vi "Supervisor MATLAB Write Client.vi"() -> ()   [LabVIEW 2017]
uses:
  <vilib>/OPCUA/controls/Write Status.ctl
  <vilib>/OPCUA/controls/NodeId.ctl
  <vilib>/OPCUA/client/Multiple Write Bool Array.vi
  <vilib>/OPCUA/NI OPC UA Client.lvlib
panel:
  in  "error in (no error)":errorcluster
  in  "Stop MATLAB Control":bool
  in  "Node Status":T1 items=["Good"=0, "Uncertain_InitialValue"=1083310080, "Uncertain_LastUsableValue"=1083179008, "Uncertain_SensorNotAccurate"=1083375616, "Uncertain_EngineeringUnitsExceeded"=1083441152, "Bad_NoCommunication"=2150694912, "Bad_NotReadable"=2151284736, "Bad_NotWritable"=2151350272, "Bad_OutOfRange"=2151415808, "Bad_WaitingForInitialData"=2150760448]
  in  "Time Stamp":timestamp
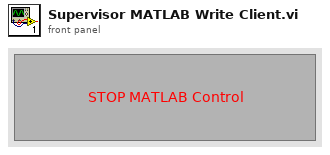
[diagram p1: front panel]
types:
  T1 = typedef "Write Status.ctl" = u32
  T2 = cluster{"message mode":enum16{"None", "Sign", "Sign and Encrypt"}, "security":enum16{"Basic256", "Basic128Rsa15"}}
  T3 = typedef "OPC UA Client Refnum.ctl" = refnum<k21>
  T4 = typedef "NodeId.ctl" = string
  T5 = cluster{"node ID":T4, "value":bool[], "timestamp (current time)":timestamp, "node status":T1}
  T6 = cluster{"node ID":T4, "value":bool[], "timestamp (current time)":timestamp, "node status":T1}[]
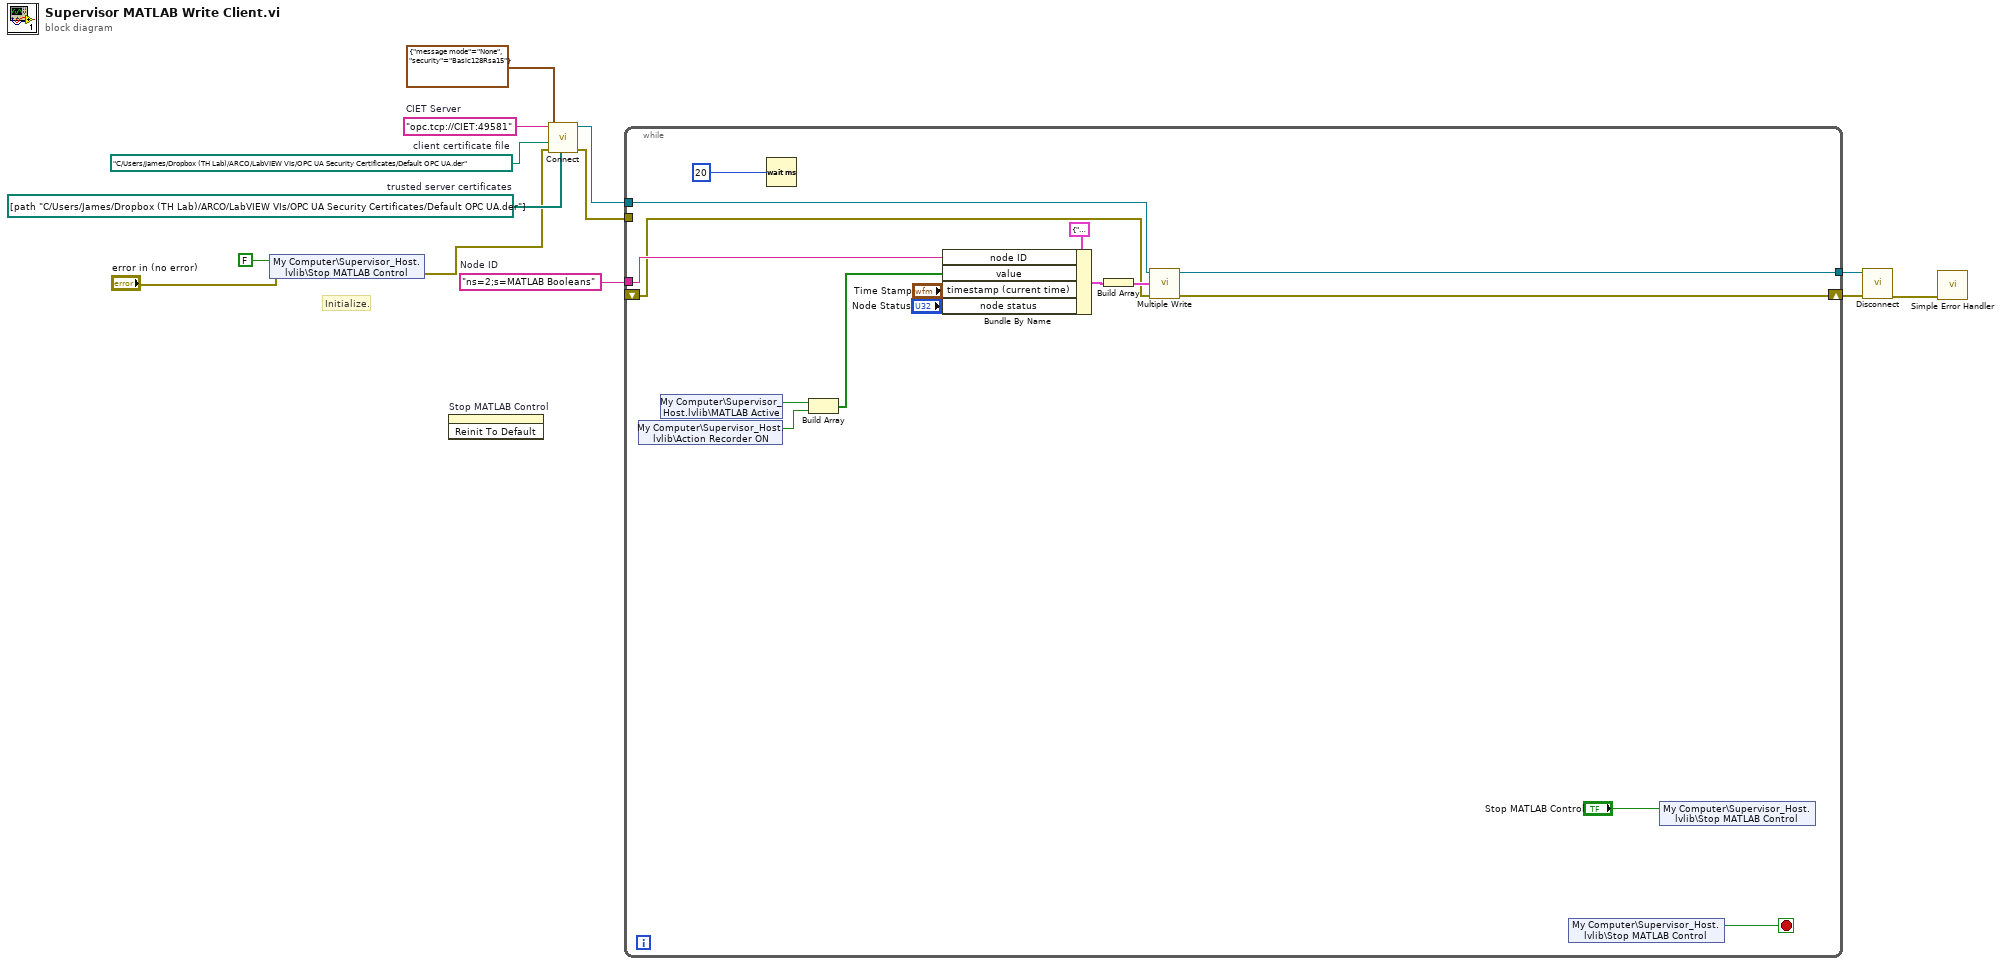
[diagram p0: block diagram]
diagram:
  w9 = "ns=2;s=MATLAB Booleans"  # Node ID
  w10 = path[] [path "C:/Users/James/Dropbox (TH Lab)/ARCO/LabVIEW VIs/OPC UA Security Certificates/Default OPC UA.der"]  # trusted server certificates
  w11 = path "C:/Users/James/Dropbox (TH Lab)/ARCO/LabVIEW VIs/OPC UA Security Certificates/Default OPC UA.der"  # client certificate file
  w13 = "opc.tcp://CIET:49581"  # CIET Server
  # "Initialize."
  n1 = shared-variable "My Computer\\Supervisor_Host.lvlib\\Stop MATLAB Control"(FALSE ("Stop MATLAB Control"), error in="error in (no error)") -> (error out=w2:errorcluster)
  n2 = invoke on="Stop MATLAB Control" class="Bool (strict)" method="Reinit To Default"() -> ()  [unwired: 3 in, 3 out]
  n3 = call <vilib>:"Connect.vi"("trusted server certificates"=w10, "error in (no error)"=w2, "client certificate file"=w11, "security policy"=T2 {"message mode"=enum."None", "security"=enum."Basic128Rsa15"}, "server endpoint URL"=w13) -> ("error out"=w8:errorcluster, "OPC UA client refnum out"=w7:T3)  [unwired: 4 in, 1 out]
  n4 = while {
    tunnel: w9 -> [w25]
    tunnel: w8 -> [_]
    tunnel: w7 -> [w19]
    tunnel: [w18] -> w5
    shift-right: [w17] -> w4
    shift-left: _ -> [w16]
    stop <- w14 stop-if-true
    n5 = shared-variable "My Computer\\Supervisor_Host.lvlib\\Action Recorder ON"() -> (w27:bool)  [unwired: 1 in, 1 out]
    n6 = shared-variable "My Computer\\Supervisor_Host.lvlib\\MATLAB Active"() -> (w28:bool)  [unwired: 1 in, 1 out]
    n7 = Wait (ms)(milliseconds to wait=u32 20) -> ()  [unwired: 1 out]
    n8 = Build Array(w28, w27) -> (w26:bool[])
    n9 = Bundle By Name(cluster=T5 {"node ID"="", "value"=[], "timestamp (current time)"=timestamp(0 s since 1904-01-01), "node status"=0} ("request"), "node ID"=w25, "value"=w26, "timestamp (current time)"="Time Stamp", "node status"="Node Status") -> (w21:T5)
    n10 = Build Array(w21) -> (w20:T6)
    n11 = call-poly <vilib>:"Multiple Write.vi"("error in (no error)"=w16, "requests"=w20, "OPC UA client refnum in"=w19) -> ("error out"=w17:errorcluster, "OPC UA client refnum out"=w18:T3)  [unwired: 5 in, 2 out]
    n12 = shared-variable "My Computer\\Supervisor_Host.lvlib\\Stop MATLAB Control"() -> (w14:bool)  [unwired: 1 in, 1 out]
    n13 = shared-variable "My Computer\\Supervisor_Host.lvlib\\Stop MATLAB Control"("Stop MATLAB Control") -> ()  [unwired: 1 in, 1 out]
  }
  n14 = call <vilib>:"Disconnect.vi"("error in (no error)"=w4, "OPC UA client refnum in"=w5) -> ("error out"=w6:errorcluster)  [unwired: 9 in]
  n15 = call <vilib>:"Simple Error Handler.vi"("error in (no error)"=w6) -> ()  [unwired: 4 in, 5 out]
